vi "Pasco_Harvester.vi"(11 "HarvClustIn":T1 {"HarvPOTElev" scale=0.0..5.0; "HarvManualElev" scale=-1.0..1.0; "HarvRollerBDesSpd" scale=-1.0..1.0; "HarvRollerFDesSpd" scale=-1.0..1.0}) -> (3 "HarvClustOut":T2 {"HarvOutRollerB" scale=-1.0..1.0; "HarvOutRollerF" scale=-1.0..1.0; "HarvOutElev" scale=-1.0..1.0})   [LabVIEW 2012]
panel:
  in  "HarvConstArrayElev":dbl[](array[numeric])=[0.0, 1.0, 2.0, 3.0, 4.0]
  in  "Harvester Speed Multiplier":dbl=0.75
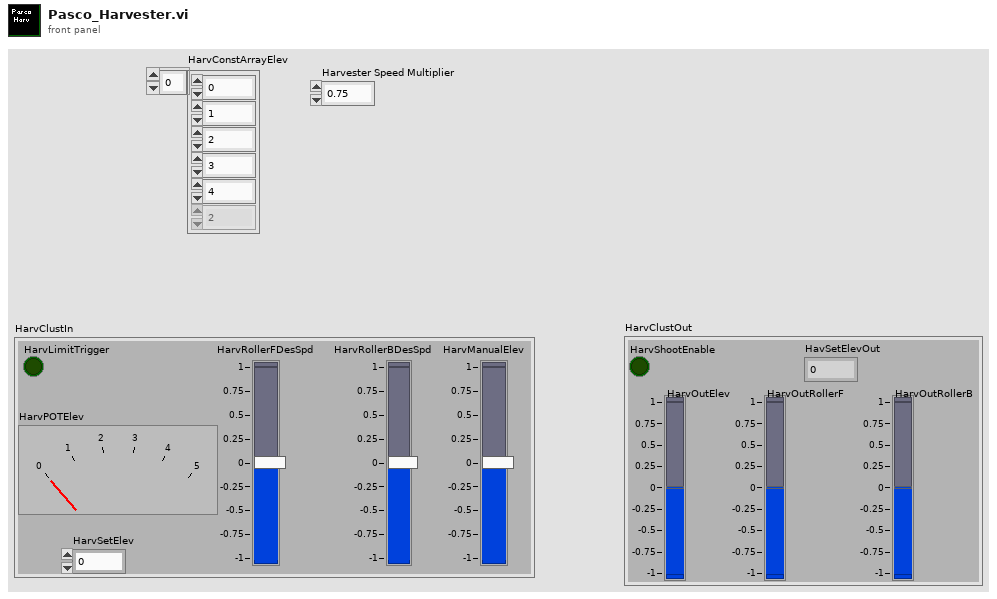
[diagram p1: front panel]
types:
  T1 = cluster{"HarvLimitTrigger":bool, "HarvRollerFDesSpd":dbl, "HarvRollerBDesSpd":dbl, "HarvManualElev":dbl, "HarvPOTElev":dbl, "HarvSetElev":i32}
  T2 = cluster{"HarvOutElev":dbl, "HarvShootEnable":bool, "HarvOutRollerF":dbl, "HarvOutRollerB":dbl, "HavSetElevOut":i32}
  T3 = cluster{"HarvOutElev":dbl, bool, "t":dbl, "t":dbl, "f":i32}
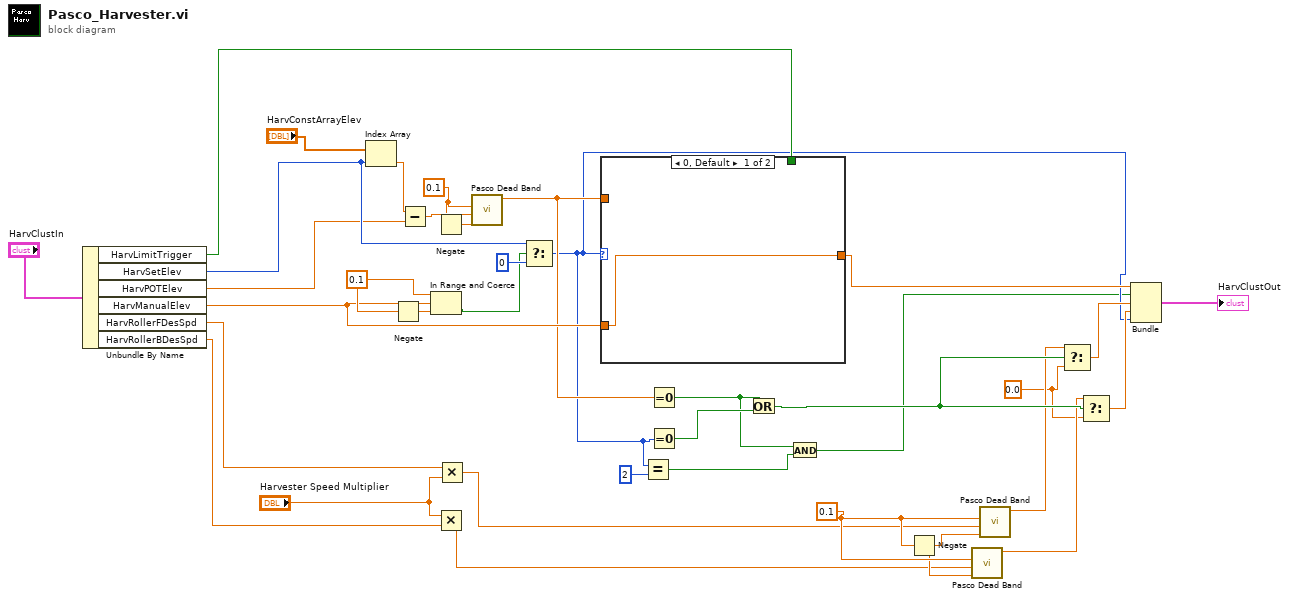
[diagram p0: block diagram]
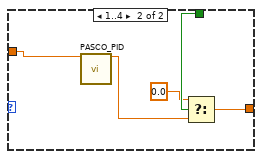
[diagram p2: hidden frame]
diagram:
  w2 = 0.0 ("t")
  w19 = 0.1 ("upper limit")
  w29 = 0.1 ("upper limit")
  w33 = 0.1 ("upper limit")
  n1 = Unbundle By Name("HarvClustIn") -> ("HarvLimitTrigger"=w20:bool, "HarvSetElev"=w26:i32, "HarvPOTElev"=w25:dbl, "HarvManualElev"=w24:dbl, "HarvRollerFDesSpd"=w23:dbl, "HarvRollerBDesSpd"=w22:dbl)
  n2 = Index Array(array="HarvConstArrayElev", index=w26) -> (element=w36:dbl)
  n3 = Negate(x=w29) -> (-x=w30:dbl)
  n4 = Subtract(x=w36, y=w25) -> (x-y=w34:dbl)
  n5 = In Range and Coerce(upper limit=w29, x=w24, lower limit=w30) -> (In Range?=w14:bool)  [unwired: 1 out]
  n6 = Negate(x=w33) -> (-x=w32:dbl)
  n7 = Multiply(x="Harvester Speed Multiplier", y=w22) -> (x*y=w9:dbl)
  n8 = Multiply(x=w23, y="Harvester Speed Multiplier") -> (x*y=w10:dbl)
  n9 = call "Pasco Dead Band.vi"("lower limit"=w32, "PWM Power"=w34, "upper limit"=w33) -> ("PWM Power"=w15:dbl)  [unwired: 7 in, 1 out]
  n10 = Select(t=w26, s=w14, f=0) -> (s? t:f=w8:i32)
  n11 = case shown="0, Default" w8 {
    tunnel: w15 -> [_ w42]
    tunnel: w24 -> [w37 _]
    tunnel: [w37 w41] -> w21
    tunnel: w20 -> [_ w39]
    frame 0, Default {
    }
    frame 1..4 {
      n12 = call "PASCO_PID.vi"("Delta"=w42) -> ("HarvOutElev"=w40:dbl)  [unwired: 14 in]
      n13 = Select(t=0.0, s=w39, f=w40) -> (s? t:f=w41:dbl)
    }
  }
  n14 = Equal?(x=w8, y=2) -> (x = y?=w6:bool)
  n15 = Equal To 0?(x=w15) -> (x = 0?=w1:bool)
  n16 = Equal To 0?(x=w8) -> (x = 0?=w11:bool)
  n17 = Or(x=w1, y=w11) -> (x .or. y?=w12:bool)
  n18 = And(x=w1, y=w6) -> (x .and. y?=w5:bool)
  n19 = Negate(x=w19) -> (-x=w18:dbl)
  n20 = call "Pasco Dead Band.vi"("lower limit"=w18, "PWM Power"=w9, "upper limit"=w19) -> ("PWM Power"=w3:dbl)  [unwired: 7 in, 1 out]
  n21 = call "Pasco Dead Band.vi"("lower limit"=w18, "PWM Power"=w10, "upper limit"=w19) -> ("PWM Power"=w4:dbl)  [unwired: 7 in, 1 out]
  n22 = Select(t=w4, s=w12, f=w2) -> (s? t:f=w17:dbl)
  n23 = Select(t=w3, s=w12, f=w2) -> (s? t:f=w16:dbl)
  n24 = Bundle("HarvOutElev"=w21, w5, "t"=w17, "t"=w16, "f"=w8) -> (→"HarvClustOut":T3)  [unwired: 1 in]
